vi "Send Delayed Device Activate.vi"(4 "Milliseconds To Wait":i32=1000, 6 "Activate Mode":T1, 7 "Message Priority (Normal)":T2=enum."Normal", 8 "error in (no error)":errorcluster, 10 "IED Name":string, 11 "Message Enqueuer":refnum<class "Message Enqueuer.lvclass">) -> (0 "error out":errorcluster)   [LabVIEW 2015, in "SCADA Core.lvlib" / "Device Activate Msg.lvclass"]
doc: "This VI sends the message to an actor."
uses:
  Device Activate Msg.lvclass
  <vilib>/ActorFramework/Message Enqueuer/Message Enqueuer.lvclass
  <vilib>/ActorFramework/Message Enqueuer/Message Priority.ctl
  IED Actor/IED/Controls/Device Activate Mode Select.ctl
  Device Activate Msg.lvclass/Device Activate Msg.ctl
  IED Actor/IED/IED.lvclass
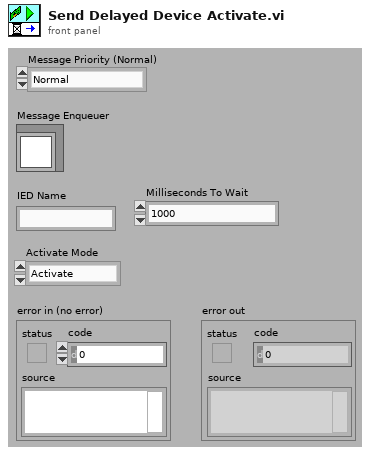
[diagram p1: front panel]
types:
  T1 = typedef "IED Actor.lvlib/IED.lvclass/Device Activate Mode Select.ctl" = enum16{"Activate", "Blackstart", "Individual"}
  T2 = typedef "Actor Framework.lvlib/Message Enqueuer.lvclass/Message Priority.ctl" = enum16{"Low", "Normal", "High"}
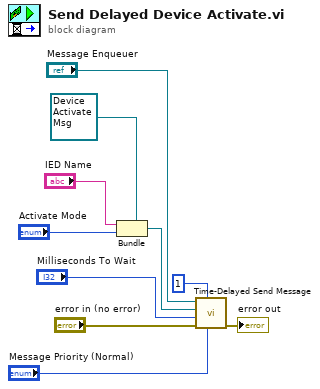
[diagram p0: block diagram]
diagram:
  n1 = Bundle(cluster=refnum<class "Device Activate Msg.lvclass"> refnum ("Object"), "IED Name", "Activate Mode") -> (w6:refnum<class "Device Activate Msg.lvclass">)
  n2 = call <vilib>:"Time-Delayed Send Message.vi"("Message Priority (Normal)"="Message Priority (Normal)", "# Copies (0 = infinite repeat)"=u32 1, "error in (no error)"="error in (no error)", "Milliseconds To Wait"="Milliseconds To Wait", "Message"=w6, "Message Enqueuer"="Message Enqueuer") -> ("error out"=→"error out":errorcluster)  [unwired: 4 in, 1 out]
